vi "Save All.vi"(8 "error in (no error)":errorcluster, 11 "Rename in":refnum<class "ProjectItem.lvclass">) -> (0 "error out":errorcluster, 3 "Rename out":refnum<class "ProjectItem.lvclass">)   [LabVIEW 2019, in "ProjectItem.lvclass"]
uses:
  ProjectItem.lvclass
  ProjectItem.lvclass/ProjectItem.ctl
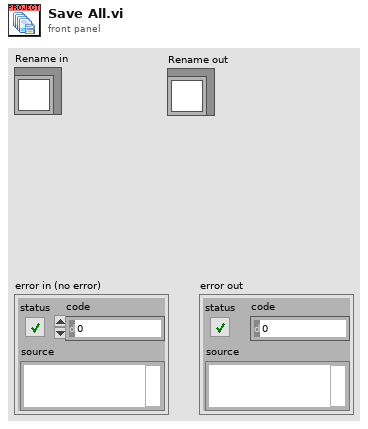
[diagram p1: front panel]
types:
  T1 = cluster{"Class":refnum<vi>, "DynamicVIs":refnum<vi>[], "StaticVIs":refnum<vi>[], "Controls":refnum<vi>[], "Name":string, "Icon":refnum<class "Icon.lvclass">, "Wire Foreground Color":u32}[]
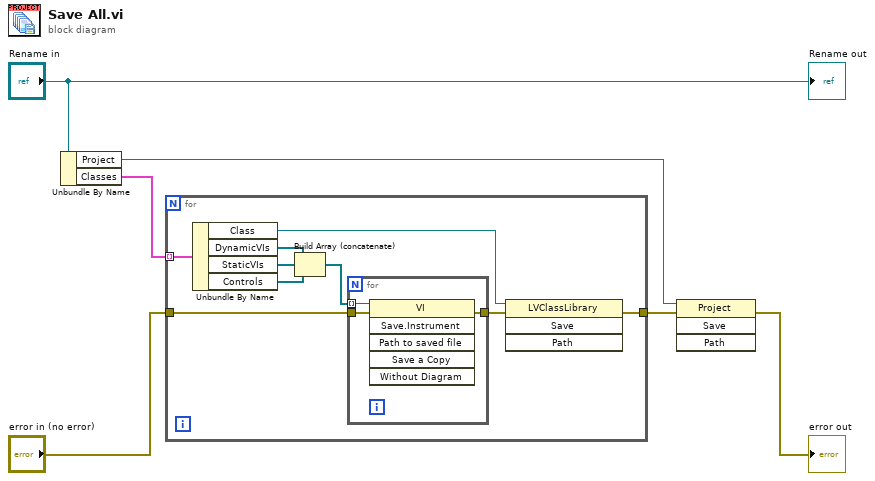
[diagram p0: block diagram]
diagram:
  n1 = Unbundle By Name("Rename in") -> ("Project"=w5:refnum<vi>, "Classes"=w1:T1)
  n2 = for {
    tunnel: w1 -> [w15] mode=indexing
    tunnel: "error in (no error)" -> [w11]
    tunnel: [w8] -> w4
    n3 = Unbundle By Name(w15) -> ("Class"=w9:refnum<vi>, "DynamicVIs"=w13:refnum<vi>[], "StaticVIs"=w14:refnum<vi>[], "Controls"=w7:refnum<vi>[])
    n4 = Build Array (concatenate)(w13, w14, w7) -> (w12:refnum<vi>[])
    n5 = for {
      tunnel: w12 -> [w18] mode=indexing
      tunnel: w11 -> [w17]
      tunnel: [w16] -> w10
      n6 = invoke class="VI" method="Save.Instrument"(reference=w18, error in=w17) -> (error out=w16:errorcluster)  [unwired: 4 in, 5 out]
    }
    n7 = invoke class="LVClassLibrary" method="Save"(reference=w9, error in=w10) -> (error out=w8:errorcluster)  [unwired: 2 in, 3 out]
  }
  n8 = invoke class="Project" method="Save"(reference=w5, error in=w4) -> (error out=→"error out":errorcluster)  [unwired: 2 in, 3 out]
  "Rename out" <- "Rename in"
